vi "TDT-Write AO2.vi"(0 "RPcox":refnum<k7>, 5 "Next Buffer":i32, 7 "Input array":dbl[][](array[numeric]), 9 "Chans":i32[](array[numeric]), 11 "error in (no error)":errorcluster) -> (4 "RPcox (thru)":refnum<k7>, 15 "error out":errorcluster)   [LabVIEW 2015]
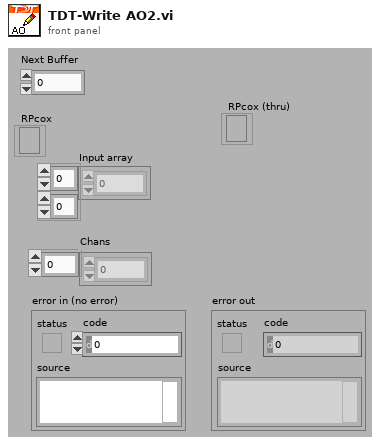
[diagram p1: front panel]
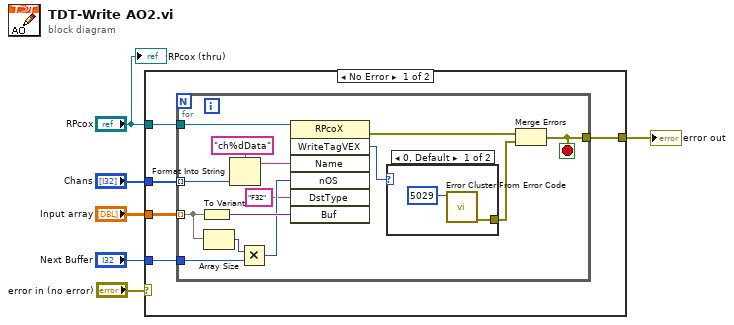
[diagram p0: block diagram]
diagram:
  n1 = case shown="No Error" "error in (no error)" {
    selector: "error in (no error)" -> [_ w28]
    tunnel: "Next Buffer" -> [w11 _]
    tunnel: "Input array" -> [w10 _]
    tunnel: "RPcox" -> [w9 _]
    tunnel: [w8 w28] -> w2
    tunnel: "Chans" -> [w7 _]
    frame No Error {
      n2 = for {
        tunnel: w9 -> [w25]
        tunnel: w10 -> [w16] mode=indexing
        tunnel: [w14] -> w8
        tunnel: w11 -> [w21]
        tunnel: w7 -> [w12] mode=indexing
        stop <- w14 stop-if-true
        n3 = To Variant(anything=w16) -> (Variant=w20:variant)
        n4 = Array Size(array=w16) -> (size(s)=w17:i32)
        n5 = Format Into String(format string="ch%dData", w12) -> (resulting string=w23:string)  [unwired: 2 in, 1 out]
        n6 = Multiply(x=w17, y=w21) -> (x*y=w19:i32)
        n7 = invoke class="RPcoX" method="WriteTagVEX"(reference=w25, "Name"=w23, "nOS"=w19, "DstType"="F32", "Buf"=w20) -> (error out=w22:errorcluster, "WriteTagVEX"=w15:i32)  [unwired: 2 in, 5 out]
        n8 = case shown="0, Default" w15 {
          tunnel: [w26 _] -> w13
          frame 0, Default {
            n9 = call <vilib>:"Error Cluster From Error Code.vi"("error code (0)"=5029) -> ("error out"=w26:errorcluster)  [unwired: 8 in]
          }
          frame 1 {
          }
        }
        n10 = Merge Errors(w22, w13) -> (w14:errorcluster)
      }
    }
    frame Error {
    }
  }
  "error out" <- w2
  "RPcox (thru)" <- "RPcox"
